vi "AVI-Load playback parameters.vi"(8 "error in (no error)":errorcluster, 9 "AVI File Path":path=path "D:/Microscope data/10 Sep 2014/TimeLapse 10_09_2014 18-46-40 512x512/Experiment Header.ini", 11 "I16 image ref":T1) -> (0 "error out":errorcluster)   [LabVIEW 2013]
uses:
  <vilib>/vision/Image Controls.llb/IMAQ Image.ctl
  Functional Imaging Viewer/SubVIs/Experiment header interface/Typedefs/Header file type enum.ctl
  Functional Imaging Viewer/SubVIs/Experiment header interface/Typedefs/Header file interface module functions enum.ctl
  Globals/gl_Time series viewer globals.vi
  Global Variables/General Globals.vi
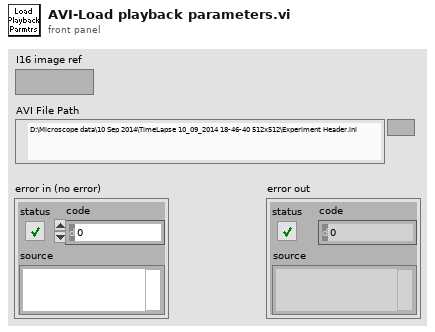
[diagram p1: front panel]
types:
  T1 = typedef "IMAQ Image.ctl" = refnum<image>
  T2 = typedef "Header file interface module functions enum.ctl" = enum16{"Load experiment header file", "Save experiment header file", "Clear stored values", "Read stored values", "Update specific value in memory", "Update all values in memory"}
  T3 = typedef "Header file type enum.ctl" = enum16{"All parameters", "Params for funct acq w ROI or mscn", "Params for funct acq w rectangles", "Live imaging header parameters", "AOL Parameters"}
  T4 = typedef "Header parameters cluster-ALL.ctl" = cluster{"Imaging Protocol":T5, "Number of POI":u16, "Number of Miniscans":u16, "Number of Trials":u16, "Number of Cycles ":u64, "# Averaged Frames":u16, "Laser power (%)":u8, "Pockels":dbl, "Acquisition Length (sec)":dbl, "Fill time (us)":dbl, "POI Dwell time (us)":dbl, "Miniscan Dwell time per pixel (us)":dbl, "PMT 1":dbl, "PMT 2":dbl, "Back Apperture":dbl, "Zoom":dbl, "Frame Size":T6, "Center Frequency":dbl, "Field of View":dbl, "DwellTime (us)":dbl, "Wavelength (nm)":dbl, "AOL Z":dbl, "AOL Mode":T7, "GridXY":dbl, "GridZ":dbl, "TriggerDelay (sec)":dbl, "Number of Pixels in Miniscan":u16, "Experiment folder path":path, "X centre":dbl, "Y centre":dbl, "Angle (degrees)":dbl, "Plane Mode":T8, "Software version":dbl, "Objective":T9, "MotorZ Calibration":u32, "Pockels Calibration":u32, "Threshold":u16[], "Video length (sec)":dbl, "Frame rate (fps)":u8, "Rectangle ROI length (pixels)":u16, "Rectangle ROI height (pixels)":u16}
  T5 = typedef "Imaging Protocols enum.ctl" = enum16{"AOL Z-Stack", "Motor Z Stack", "Functional Acquisition", "Single Plane Acquisition", "Volume Acquisition", "Live Imaging", "Live Plane Imaging", "Live Volume Imaging"}
  T6 = typedef "Frame Size.ctl" = u16
  T7 = typedef "AOL modes.ctl" = enum16{"Raster", "Structural", "Pointing", "Mini Scan", "Alignment"}
  T8 = typedef "Plane Mode.ctl" = u16
  T9 = typedef "Objective selector control enum.ctl" = string
  T10 = typedef "AVI playback header info cluster.ctl" = cluster{"Frame Size":u32, "AOD fill time (us)":dbl, "Dwell time (us)":dbl, "Frame period (ms)":dbl, "Number of Miniscans":u16, "Number of Pixels in Miniscan":u16}
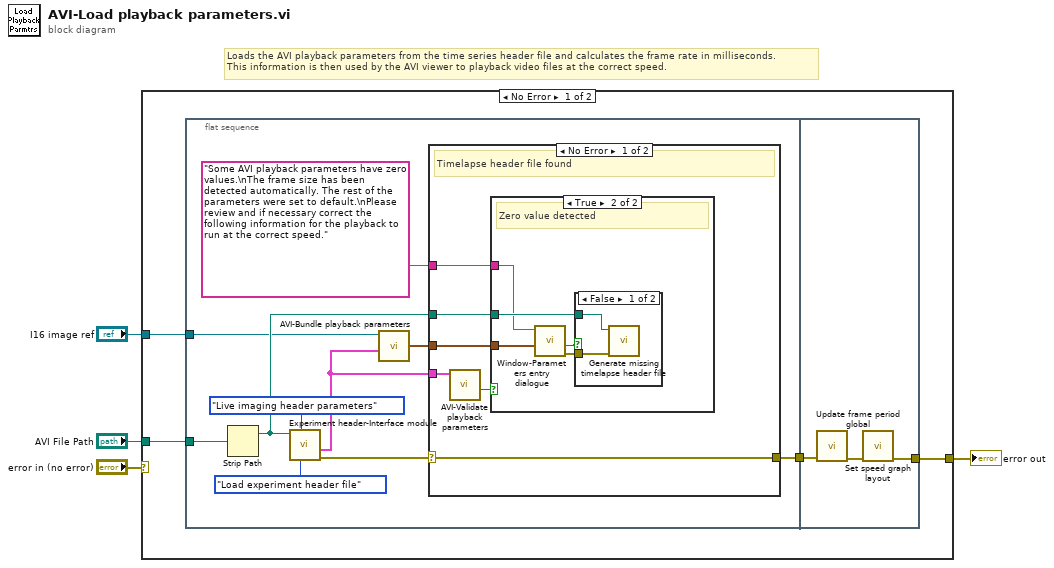
[diagram p0: block diagram]
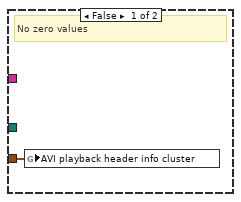
[diagram p2: hidden frame]
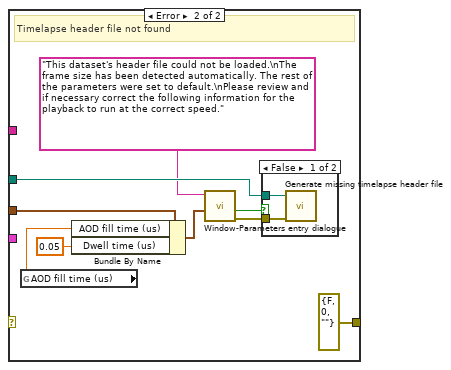
[diagram p4: hidden frame]
diagram:
  # "Loads the AVI playback parameters from the time series header file and calculates the frame rate in milliseconds.\nThis information is then used by the AVI viewer to playback video files at the correct speed."
  n1 = case shown="No Error" "error in (no error)" {
    selector: "error in (no error)" -> [_ w47]
    tunnel: [w6 w47] -> w4
    tunnel: "AVI File Path" -> [w8 _]
    tunnel: "I16 image ref" -> [w5 _]
    frame No Error {
      n2 = flat-sequence {
        tunnel: w8 -> [w18]
        tunnel: [w9] -> w7
        tunnel: w5 -> [w11]
        tunnel: [w44] -> w6
        tunnel: w7 -> [w46]
        frame #0 {
          n3 = Strip Path(path=w18) -> (stripped path=w14:path)  [unwired: 1 out]
          n4 = call "Experiment header-Interface module.vi"("Header file type"=Header_file_type_enum."Live imaging header parameters", "Function"=Header_file_interface_module_functions_enum."Load experiment header file", "Experiment data folder path"=w14) -> ("error out"=w15:errorcluster, "All header parameters out"=w12:T4)  [unwired: 7 in]
          n5 = call "AVI-Bundle playback parameters.vi"("All header parameters in"=w12, "I16 image ref"=w11) -> ("AVI playback header info cluster"=w13:T10)  [unwired: 9 in]
          n6 = case shown="No Error" w15 {
            selector: w15 -> [w19 _]
            tunnel: w12 -> [w23 _]
            tunnel: w14 -> [w21 w40]
            tunnel: w13 -> [w22 w36]
            tunnel: "Some AVI playback parameters have zero values.\nThe frame size has been detected automatically. The rest of the parameters were set to default.\nPlease review and if necessary correct the following information for the playback to run at the correct speed." ("Message") -> [w20 _]
            tunnel: [w19 errorcluster {"status"=FALSE, "code"=0, "source"=""} ("error IO")] -> w9
            frame No Error {
              # "Timelapse header file found"
              n7 = call "AVI-Validate playback parameters.vi"("All header parameters in"=w23) -> ("Zero value detected"=w24:bool)  [unwired: 9 in, 1 out]
              n8 = case shown="True" w24 {
                tunnel: w22 -> [w25 w29]
                tunnel: w21 -> [_ w28]
                tunnel: w20 -> [_ w26]
                frame False {
                  # "No zero values"
                  n9 = global write "gl_Time series viewer globals.vi" "AVI playback header info cluster"(w25) -> ()
                }
                frame True {
                  # "Zero value detected"
                  n10 = call "Window-Parameters entry dialogue.vi"("AVI playback header info cluster"=w29, "Message"=w26) -> ("error out"=w30:errorcluster, "Cancelled"=w27:bool)  [unwired: 8 in]
                  n11 = case shown="False" w27 {
                    tunnel: w30 -> [w32 _]
                    tunnel: w28 -> [w31 _]
                    frame False {
                      n12 = call "Generate missing timelapse header file.vi"("error in (no error)"=w32, "Timelapse data folder path"=w31) -> ()  [unwired: 10 in]
                    }
                    frame True {
                    }
                  }
                }
              }
            }
            frame Error {
              # "Timelapse header file not found"
              n13 = global read "General Globals.vi" "AOD fill time (us)"() -> (w34:dbl)
              n14 = Bundle By Name(cluster=w36, "AOD fill time (us)"=w34, "Dwell time (us)"=0.05) -> (w37:T10)
              n15 = call "Window-Parameters entry dialogue.vi"("AVI playback header info cluster"=w37, "Message"="This dataset's header file could not be loaded.\nThe frame size has been detected automatically. The rest of the parameters were set to default.\nPlease review and if necessary correct the following information for the playback to run at the correct speed.") -> ("error out"=w41:errorcluster, "Cancelled"=w38:bool)  [unwired: 8 in]
              n16 = case shown="False" w38 {
                tunnel: w41 -> [w43 _]
                tunnel: w40 -> [w42 _]
                frame False {
                  n17 = call "Generate missing timelapse header file.vi"("error in (no error)"=w43, "Timelapse data folder path"=w42) -> ()  [unwired: 10 in]
                }
                frame True {
                }
              }
            }
          }
        }
        frame #1 {
          n18 = call "Update frame period global.vi"("error in (no error)"=w46) -> ("error out"=w45:errorcluster)  [unwired: 10 in]
          n19 = call "Set speed graph layout.vi"("error in (no error)"=w45) -> ("error out"=w44:errorcluster)  [unwired: 10 in]
        }
      }
    }
    frame Error {
    }
  }
  "error out" <- w4
